vi "Acq Fetch Waveform (I16).vi"(0 "session in":refnum<class "Digitizer Control.lvclass">, 2 "elements to read":u32, 5 "error in (no error)":errorcluster, 7 "timeout (ms)":i32=5000, 8 "channel index":i32, 9 "clear time out error? (F)":bool) -> (13 "timed out?":bool, 14 "session out":refnum<class "Digitizer Control.lvclass">, 15 "sample data":i16[](array[numeric]), 17 "elements remaining":u32, 19 "error out":errorcluster)   [LabVIEW 2021, in "Digitizer Control.lvclass"]
doc: "Fetches the acquired sample data as an array of I16s. Use the <B>Acq Configure Channel.vi</B> to configure the channel parameters, the <B>Acq Configure Transfer.vi</B> to configure the waveform transfer, and the <B>Acq Configure Start Trigger.vi</B> to configure the start trigger, then use the <B>Acq Initiate.vi</B> to initiate the acquisition. After the acquisition is initiated, use this VI to fetch the acquired sample data. Use the <B>Acq Get Status.vi</B> to check the acquisition status and the <B>Acq Stop.vi</B> to stop an acquisition.\n\nInputs:\n\n<B>session in</B>: The device session.\n\n<B>channel index</B>: The index of the channel to read.\n\n<B>elements to read</B>: The number of elements to read from the host DMA buffer to fetch the acquired sample data. For example, in case of a finite acquisition wire the <B>elements to read</B> output of the <B>Acq Initiate.vi</B> to this input.\n\n<B>timeout</B>: The maximum amount of time, in milliseconds, this VI is allowed to wait for the requested number of elements to become available.\n\n<B>clear time out error?</B>: If this input is true, then the <B>error out</B> output does not return the time out error.\n\nOutputs:\n\n<B>session out</B>: The device session passed on the <B>session in</B> input.\n\n<B>sample data</B>: The acquired sample data as an array of I16s. The samples are using fixed point representation: the size of a sample is <B>sample size (bits)</B> bits. The bits of the samples are placed in the I16 elements with LSB first bit packing. To convert the returned I16 array to samples scaled to Volts: unpack the samples then multiply the samples by <B>sample scale factor</B> * 2^-( <B>sample size (bits)</B> ), where <B>sample scale factor</B> is returned by the <B>Acq Configure Channel.vi</B>, while <B>sample size (bits)</B> is returned by the <B>Acq Configure Transfer.vi</B>.\n\n<B>elements remaining</B>: The number of additional elements remaining in the host DMA buffer that are available for reading.\n\n<B>timed out?</B>: A true on this output indicates that the fetch operation timed out.\n\nNotes:\n\nDo not mix the different Acq Fetch Waveform VIs. Once this VI is called on a channel, use only this VI to fetch the acquired samples on that channel. If you want to use another fetch VI, then it is recommended to reconfigure the transfer first using the <B>Acq Configure Transfer.vi</B>."
uses:
  Digitizer Control.lvclass
  Digitizer Control.lvclass/Digitizer Control.ctl
  <vilib>/Utility/error.llb/Error Cluster From Error Code.vi
  <vilib>/rvi/errors/niLvFpgaAdjustHostInterfaceError.vi
  <vilib>/rvi/interface/nirviMethod/nirviMethod.xnode
  <vilib>/ErrorRing/Error Ring.xnode
  <vilib>/FPGAPlugInAG/Dynamic/niLvFpga_ReadFifo_Dynamic.vi
  <vilib>/rvi/errors/niLvFpgaMergeErrorWithErrorCode.vi
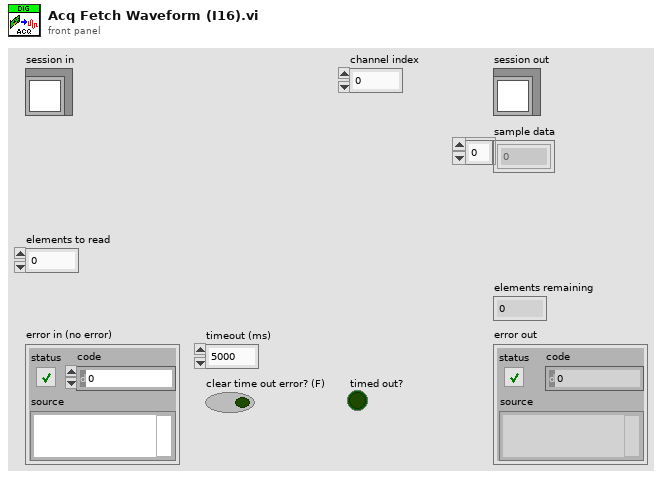
[diagram p1: front panel]
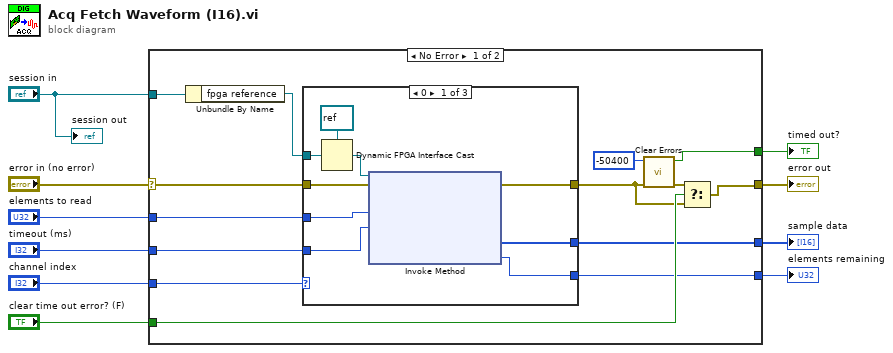
[diagram p0: block diagram]
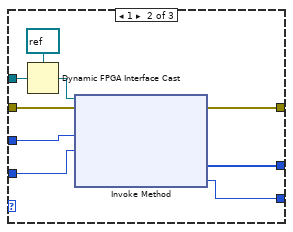
[diagram p2: hidden frame]
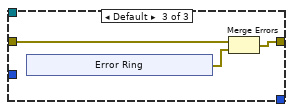
[diagram p3: hidden frame]
diagram:
  n1 = case shown="No Error" "error in (no error)" {
    selector: "error in (no error)" -> [w18 w51]
    tunnel: "elements to read" -> [w20 _]
    tunnel: [w14 w51] -> w4
    tunnel: "timeout (ms)" -> [w23 _]
    tunnel: "session in" -> [w21 _]
    tunnel: [w22 _] -> w7
    tunnel: [w19 _] -> w5
    tunnel: "clear time out error? (F)" -> [w24 _]
    tunnel: [w12 _] -> w2
    tunnel: "channel index" -> [w11 _]
    frame No Error {
      n2 = Unbundle By Name(w21) -> ("fpga reference"=w17:refnum<k20>)
      n3 = case shown="0" w11 {
        tunnel: w23 -> [w33 w42 _]
        tunnel: [w30 w39 _] -> w22
        tunnel: w20 -> [w29 w38 _]
        tunnel: [w28 w37 _] -> w19
        tunnel: w18 -> [w27 w36 w44]
        tunnel: w17 -> [w26 w35 _]
        tunnel: [w25 w34 w43] -> w13
        frame 0 {
          n4 = Dynamic FPGA Interface Cast(Session In=refnum<k20> refnum ("Type"), Type=w26) -> (Session Out=w32:refnum<k20>)
          n5 = xnode "Invoke Method"("FPGA VI Reference In"=w32, "error in"=w27, "Number of Elements"=w29, "Timeout (ms)"=w33) -> ("error out"=w25:errorcluster, "Data"=w28:i16[], "Elements Remaining"=w30:u32)  [unwired: 1 out]
        }
        frame 1 {
          n6 = Dynamic FPGA Interface Cast(Session In=refnum<k20> refnum ("Type"), Type=w35) -> (Session Out=w41:refnum<k20>)
          n7 = xnode "Invoke Method"("FPGA VI Reference In"=w41, "error in"=w36, "Number of Elements"=w38, "Timeout (ms)"=w42) -> ("error out"=w34:errorcluster, "Data"=w37:i16[], "Elements Remaining"=w39:u32)  [unwired: 1 out]
        }
        frame Default {
          n8 = xnode "Error Ring"() -> ("error out"=w45:errorcluster)
          n9 = Merge Errors(w44, w45) -> (w43:errorcluster)
        }
      }
      n10 = call <vilib>:"Clear Errors.vi"("error in (no error)"=w13, "specific error code to clear (0: all)"=-50400) -> ("error out"=w15:errorcluster, "specific error cleared?"=w12:bool)  [unwired: 4 in]
      n11 = Select(t=w15, s=w24, f=w13) -> (s? t:f=w14:errorcluster)
    }
    frame Error {
    }
  }
  "elements remaining" <- w7
  "sample data" <- w5
  "error out" <- w4
  "timed out?" <- w2
  "session out" <- "session in"
